vi "ExADCAsync.vi"() -> ()   [LabVIEW 2010]
panel:
  in  "Intensifier":bool
  out "Pixel Time":i32
  out "Bit Depth":i32
  out "ReadOut port":i32
  out "ADC Offset":i32
  out "ADC Gain":i32
  out "ADC Speed":i32
  in  "Readout Port":i32=-1 min=-1 step=1
  in  "ADC Offset":i32=-1 min=-1 step=1
  in  "ADC Gain":i32=-1 min=-1 step=1
  in  "ADC speed":i32=-2 min=-3 step=1
  in  "Trigger Edge":u32(ring)=1 items=["N/A", "Positive (leading) edge", "Negative (falling) edge"]
  in  "Timing Mode":u32(ring)=1 items=["N/A", "Free Run/Timed", "Trigger First (PM only)", "Ext Sync/Strobed ", "Variable Exp (PM only)", "Flash Mode (PM only)"]
  in  "Temperature":dbl format="%.2f"
  in  "Exposure":dbl min=0.0 step=0.001 format="%.3f"
  in  "stop":bool
  in  "Store":bool
  out "error out":errorcluster
  in  "error in (no error)":errorcluster
  # "ExADCAsync:\nThis program shows how to use the  CameraADCset.vi\nand the CameraADCget.vi. This example allows all the \nADC settings to be set or ignored. And then displays"
  # "The following are read \nfrom camera after setting\nvalues to left.\n-1 value means it isn't \nsupported by camera."
  # "For Slowest ADC speed set this to -3\nFor Fastest ADC speed set this to -2\nTo use current ADC speed don't  hook up or use -1\notherwise put speed in as kHz"
  # "To use current gain don't hook up or set to -1"
  # "To use current gain don't hook up or set to -1"
  # "To use current gain don't hook up or set to -1"
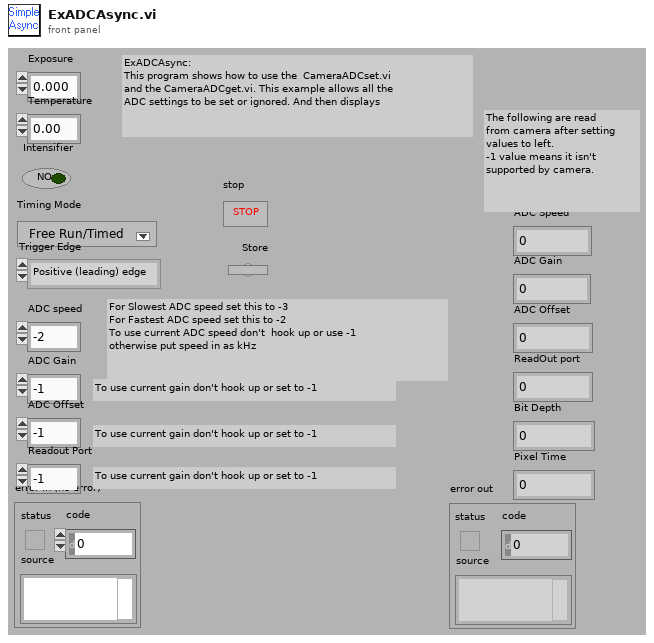
[diagram p1: front panel]
types:
  T1 = cluster{"Acquire mode \n3 is Async":i32, "Exposure":dbl, "Number of Images":i32, "Software Accums":i32}
  T2 = cluster{"Camera Handle":u32, "Pulser Handle":u32, "File Handle":u32, "Display Handle":u32, "Image Handle":u32}
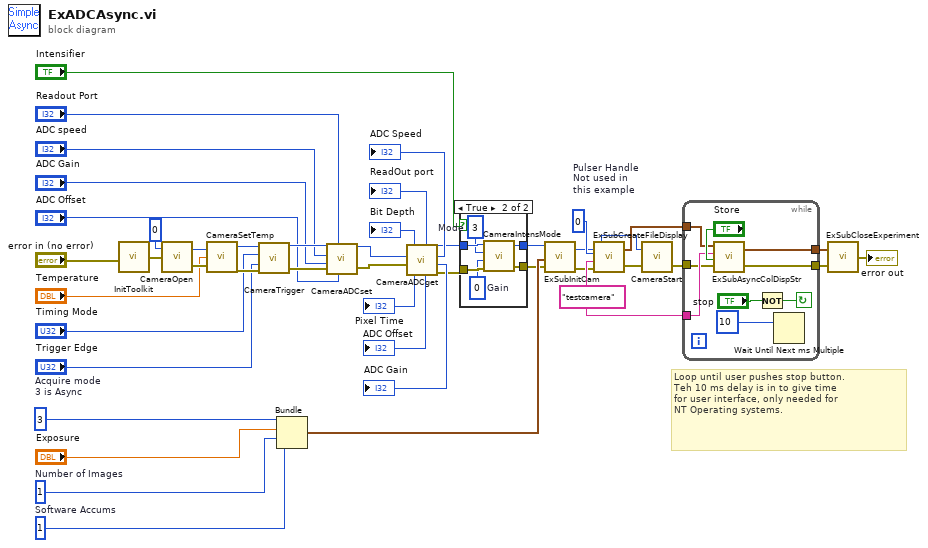
[diagram p0: block diagram]
diagram:
  w37 = 0  # Pulser Handle Not used in  this example
  w42 = 1  # Number of Images
  w43 = 3  # Acquire mode  3 is Async
  w41 = 1  # Software Accums
  w44 = "testcamera"
  # "Loop until user pushes stop button.\nTeh 10 ms delay is in to give time \nfor user interface, only needed for \nNT Operating systems."
  n1 = call <userlib>:"InitToolkit.vi"("error in"="error in (no error)") -> ("error out"=w28:errorcluster)
  n2 = call <userlib>:"CameraOpen.vi"("error in"=w28, "Camera Device ID"=0) -> ("error out"=w25:errorcluster, "Camera Handle"=w26:u32)
  n3 = call <userlib>:"CameraSetTemp.vi"("error in (no error)"=w25, "Temperature"="Temperature", "Camera Handle"=w26) -> ("error out"=w22:errorcluster, "Camera Handle"=w23:u32)
  n4 = call <userlib>:"CameraTrigger.vi"("error in"=w22, "Trigger Edge"="Trigger Edge", "Timing Mode"="Timing Mode", "Camera Handle"=w23) -> ("error out"=w10:errorcluster, "Camera Handle"=w11:u32)
  n5 = Bundle("Acquire mode \n3 is Async"=w43, "Exposure"="Exposure", "Number of Images"=w42, "Software Accums"=w41) -> (w39:T1)  [unwired: 1 in]
  n6 = call <userlib>:"CameraADCset.vi"("ADC offset"="ADC Offset", "Read Out port"="Readout Port", "error in (no error)"=w10, "ADC Gain"="ADC Gain", "ADC Speed"="ADC speed", "Camera Handle"=w11) -> ("error out"=w13:errorcluster, "Camera Handle"=w14:u32)
  n7 = call <userlib>:"CameraADCget.vi"("Camera handle"=w14, "error in (no error)"=w13) -> ("Bit Depth"=→"Bit Depth":i32, "Pixel Time"=→"Pixel Time":i32, "Readout Port"=→"ReadOut port":i32, "ADC Offset"=→"ADC Offset":i32, "Camera handle"=w2:u32, "ADC Speed"=→"ADC Speed":i32, "ADC Gain"=→"ADC Gain":i32, "error out"=w3:errorcluster)
  n8 = case shown="True" "Intensifier" {
    tunnel: w2 -> [w46 w52]
    tunnel: [w46 w51] -> w4
    tunnel: w3 -> [w45 w50]
    tunnel: [w45 w49] -> w5
    frame False {
    }
    frame True {
      w47 = u32 0  # Gain
      w48 = u32 3  # Mode
      n9 = call <userlib>:"CameraIntensMode.vi"("error in"=w50, "Intensifier Gain"=w47, "Mode"=w48, "Camera Handle"=w52) -> ("error out"=w49:errorcluster, "Camera Handle"=w51:u32)
    }
  }
  n10 = call "ExSubInitCam.vi"("error in (no error)"=w5, "Camera Information"=w39, "Camera Handle"=w4) -> ("error out"=w38:errorcluster, "Camera Handle"=w33:u32)
  n11 = call "ExSubCreateFileDisplay.vi"("error in (no error)"=w38, "File and Display Name"=w44, "Pulser Handle"=w37, "Camera Handle"=w33) -> ("error out"=w36:errorcluster, "Handles Out"=w35:T2)
  n12 = call <userlib>:"CameraStart.vi"("error in"=w36, "Camera Handle"=w33) -> ("error out"=w34:errorcluster)  [unwired: 1 out]
  n13 = while {
    tunnel: w35 -> [w59]
    tunnel: w34 -> [w57]
    tunnel: w44 -> [w58]
    tunnel: [w55] -> w31
    tunnel: [w56] -> w32
    stop <- w54 continue-if-true
    n14 = call "ExSubAsyncColDispStr.vi"("error in (no error)"=w57, "Store Data"="Store", "Display Title"=w58, "Handle Cluster"=w59) -> ("error out"=w55:errorcluster, "Handle Cluster Out"=w56:T2)
    n15 = Not(x="stop") -> (.not. x?=w54:bool)
    n16 = Wait Until Next ms Multiple(millisecond multiple=10) -> ()  [unwired: 1 out]
  }
  n17 = call "ExSubCloseExperiment.vi"("error in (no error)"=w31, "Handles In"=w32) -> ("error out"=→"error out":errorcluster)
